vi "Runner_Enter.vi"(8 "error in":errorcluster) -> (0 "error out":errorcluster, 3 "Runner's Data OUT":T1)   [LabVIEW 2025]
uses:
  Controls/Runner_Data_Structure.ctl
panel:
  in  "Runner's Data IN":T1
  in  "Button":bool
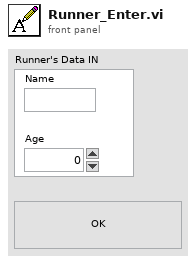
[diagram p1: front panel]
types:
  T1 = typedef "Runner_Data_Structure.ctl" = cluster{"Name":string, "Age":i32}
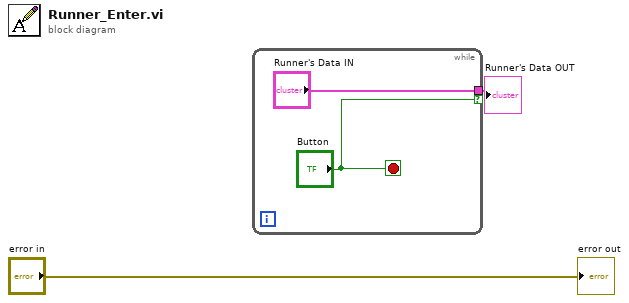
[diagram p0: block diagram]
diagram:
  n1 = while {
    tunnel: ["Runner's Data IN"] -> w1 if="Button"
    stop <- "Button" stop-if-true
  }
  "Runner's Data OUT" <- w1
  "error out" <- "error in"
